vi "Test GitHub Issues.vi"(8 "error in (no error)":errorcluster) -> (0 "error out":errorcluster)   [LabVIEW 2013]
uses:
  <vilib>/addons/_JKI Toolkits/Caraya/classes/Test/Test.lvclass
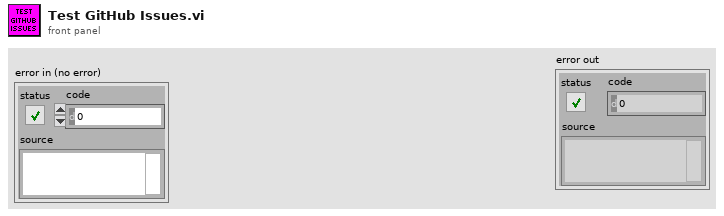
[diagram p1: front panel]
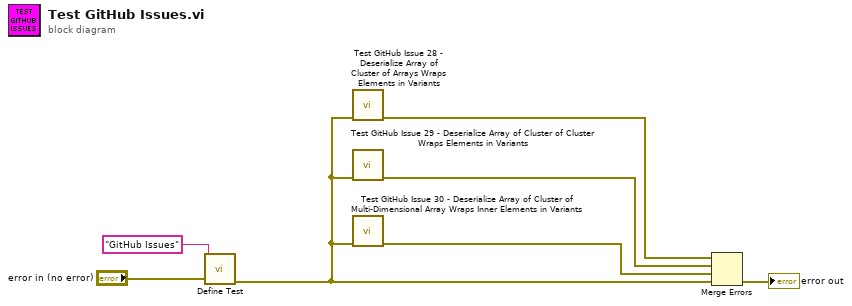
[diagram p0: block diagram]
diagram:
  n1 = call <vilib>:"Define Test.vi"("error in (no error)"="error in (no error)", "Label (VI Title)"="GitHub Issues") -> ("error out"=w2:errorcluster)  [unwired: 9 in]
  n2 = call "Test GitHub Issue 28 - Deserialize Array of Cluster of Arrays Wraps Elements in Variants.vi"("error in (no error)"=w2) -> ("error out"=w4:errorcluster)  [unwired: 10 in]
  n3 = call "Test GitHub Issue 29 - Deserialize Array of Cluster of Cluster Wraps Elements in Variants.vi"("error in (no error)"=w2) -> ("error out"=w3:errorcluster)  [unwired: 10 in]
  n4 = call "Test GitHub Issue 30 - Deserialize Array of Cluster of Multi-Dimensional Array Wraps Inner Elements in Variants.vi"("error in (no error)"=w2) -> ("error out"=w1:errorcluster)  [unwired: 10 in]
  n5 = Merge Errors(w4, w3, w1, w2) -> (→"error out":errorcluster)
